vi "LowPassSmoothing.vi"(10 "NewValueWeighting":dbl, 11 "New Value":dbl) -> (3 "Filtered Value":dbl)   [LabVIEW 2018]
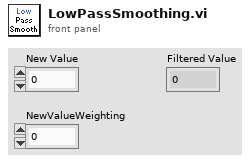
[diagram p1: front panel]
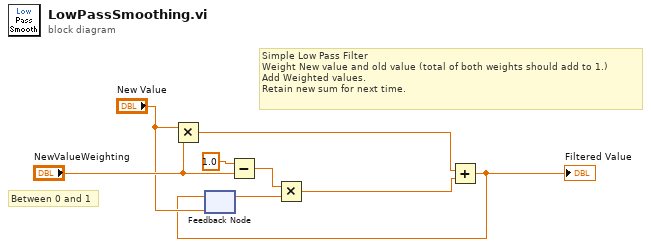
[diagram p0: block diagram]
diagram:
  # "Between 0 and 1"
  # "Simple Low Pass Filter\nWeight New value and old value (total of both weights should add to 1.)\nAdd Weighted values.\nRetain new sum for next time."
  n1 = Multiply(x="New Value", y="NewValueWeighting") -> (x*y=w8:dbl)
  n2 = feedback #1("New Value") -> (w6:dbl)
  n3 = Subtract(x=1.0 ("y"), y="NewValueWeighting") -> (x-y=w5:dbl)
  n4 = Multiply(x=w5, y=w6) -> (x*y=w7:dbl)
  n5 = Add(x=w8, y=w7) -> (x+y=w1:dbl)
  "Filtered Value" <- w1
  n6 = feedback-in #1(w1) -> ()
